vi "Up Heap.vi"(8 "error in (no error)":errorcluster, 10 "index":i32, 11 "Astar Open List in":refnum<class "NI_Robotics_Priority Queue.lvclass">) -> (0 "error out":errorcluster, 3 "Astar Open List out":refnum<class "NI_Robotics_Priority Queue.lvclass">)   [LabVIEW 2017, in "NI_Robotics_Priority Queue.lvclass"]
uses:
  <vilib>/robotics/Navigation/shared/Priority Queue/NI_Robotics_Priority Queue.lvclass
  <vilib>/robotics/Navigation/shared/Priority Queue/NI_Robotics_Priority Queue.lvclass/NI_Robotics_Priority Queue.ctl
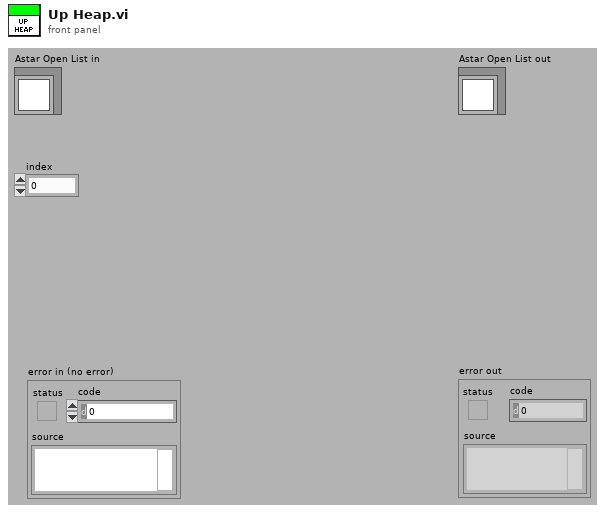
[diagram p1: front panel]
types:
  T1 = typedef "NI_Robotics_Priority Queue.lvclass/Open List Element.ctl" = cluster{"f":dbl, "g":dbl, "node Ref":refnum<data-value>}
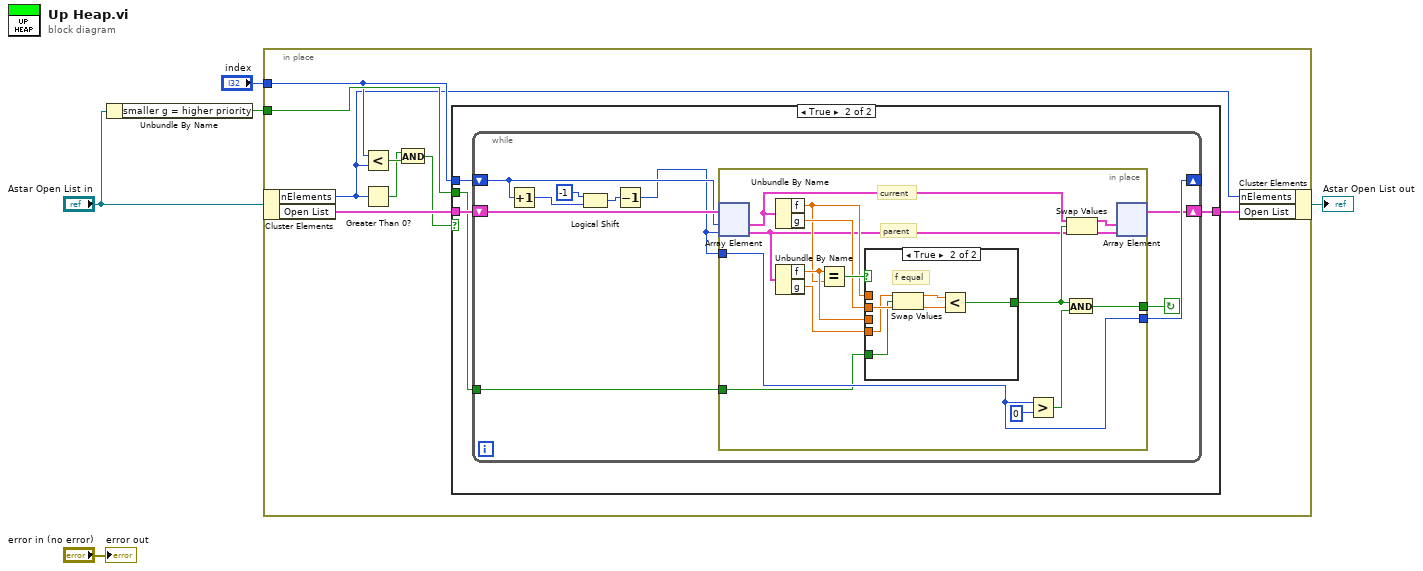
[diagram p0: block diagram]
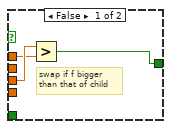
[diagram p3: hidden frame]
diagram:
  n1 = Unbundle By Name("Astar Open List in") -> ("smaller g = higher priority"=w2:bool)
  n2 = in-place {
    in-place-border: w2 -> [w12]
    in-place-border: "index" -> [w10]
    n3 = in-place-cluster #1("Astar Open List in") -> ("nElements"=w9:i32, "Open List"=w11:T1[])
    n4 = Less?(x=w10, y=w9) -> (x < y?=w8:bool)
    n5 = Greater Than 0?(x=w9) -> (x > 0?=w7:bool)
    n6 = And(x=w7, y=w8) -> (x .and. y?=w6:bool)
    n7 = case shown="True" w6 {
      tunnel: [w14 w18] -> w13
      tunnel: w11 -> [w14 w17]
      tunnel: w10 -> [_ w16]
      tunnel: w12 -> [_ w15]
      frame False {
        # "If only 1 element in the queue then do not attempt swapping"
      }
      frame True {
        n8 = while {
          shift-right: [w25] -> _
          shift-left: w16 -> [w21]
          shift-right: [w22] -> w18
          shift-left: w17 -> [w23]
          tunnel: w15 -> [w19]
          stop <- w24 continue-if-true
          n9 = Increment(x=w21) -> (x+1=w28:i32)
          n10 = Logical Shift(y=i8 -1, x=w28) -> (x << y=w26:i32)
          n11 = Decrement(x=w26) -> (x-1=w20:i32)
          n12 = in-place {
            in-place-border: [w32] -> w25
            in-place-border: [w40] -> w24
            in-place-border: w20 -> [w32]
            in-place-border: w19 -> [w29]
            # "current"
            # "parent"
            n13 = in-place-array #2(w23, w21, w20) -> (w30:T1, w31:T1)
            n14 = Unbundle By Name(w30) -> ("f"=w33:dbl, "g"=w35:dbl)
            n15 = Unbundle By Name(w31) -> ("f"=w34:dbl, "g"=w36:dbl)
            n16 = Equal?(x=w34, y=w33) -> (x = y?=w43:bool)
            n17 = case shown="True" w43 {
              tunnel: w35 -> [_ w51]
              tunnel: w36 -> [_ w50]
              tunnel: w34 -> [w45 _]
              tunnel: w33 -> [w44 _]
              tunnel: [w46 w52] -> w37
              tunnel: w29 -> [_ w47]
              frame False {
                # "swap if f bigger\nthan that of child"
                n18 = Greater?(x=w45, y=w44) -> (0:w46:bool)
              }
              frame True {
                # "f equal"
                n19 = Swap Values(12:w50, 13:w47, 14:w51) -> (1:w49:dbl, 3:w48:dbl)
                n20 = Less?(x=w49, y=w48) -> (x < y?=w52:bool)
              }
            }
            n21 = Greater?(x=w32, y=0) -> (0:w41:bool)
            n22 = And(x=w37, y=w41) -> (x .and. y?=w40:bool)
            n23 = Swap Values(12:w30, 13:w37, 14:w31) -> (1:w39:T1, 3:w38:T1)
            n24 = in-place-array #2(w39, w38) -> (w22:T1[])  [unwired: 2 out]
          }
        }
      }
    }
    n25 = in-place-cluster #1("nElements"=w9, "Open List"=w13) -> (→"Astar Open List out":refnum<class "NI_Robotics_Priority Queue.lvclass">)
  }
  "error out" <- "error in (no error)"
